vi "Compile Data Replay Loops.vi"(8 "error in (no error)":errorcluster, 10 "Channel Descriptors in":T1, 11 "Custom Device Ref":T11 format="%.0x") -> (0 "error out":errorcluster, 2 "Channel Descriptors out":T1, 3 "Custom Device Ref dup":T11 format="%.0x", 4 "DataReplayLoops":T9[](array[typedef]), 6 "DataReplayVoltages":T8[](array[typedef]))   [LabVIEW 2011, in "Engine Sim System Explorer.lvlib"]
uses:
  Engine Sim System Explorer.lvlib
  <vilib>/NI Veristand/Custom Device API/Custom Device Item Ref.ctl
  Shared/DataReplayLoopConfig.ctl
  Shared/DataReplayConfig.ctl
  Shared/DataReplayVoltageConfig.ctl
  Shared/Channel Descriptors.ctl
  Shared/FPGA Write Descriptor.ctl
  Shared/InputChannelTypes.ctl
  <vilib>/rvi/DataTransferAndStorage/Container/Common/niFpgaDataTypeControl.ctl
  Shared/FPGA Read Descriptor.ctl
  Shared/OutputChannelTypes.ctl
  Shared/Status Chan Descriptor.ctl
  Shared/Engine Simulation Global.vi
  <vilib>/NI Veristand/Custom Device Tools/Custom Device Utility Library/NI VeriStand - Search for All Items by GUID.vi
  <vilib>/NI Veristand/Custom Device API/Get Item Property (Double).vi
  <vilib>/rvi/Analysis/host/Private/Sample Rate To Loop Time (ticks).vi
  <vilib>/NI Veristand/Custom Device Tools/Custom Device Utility Library/Custom Device Utility Library.lvlib
  Engine Simulation Shared.lvlib
  <vilib>/rvi/Analysis/host/Public/NI_FpgaMspHost.lvlib
  <vilib>/NI Veristand/Custom Device API/Custom Device API.lvlib
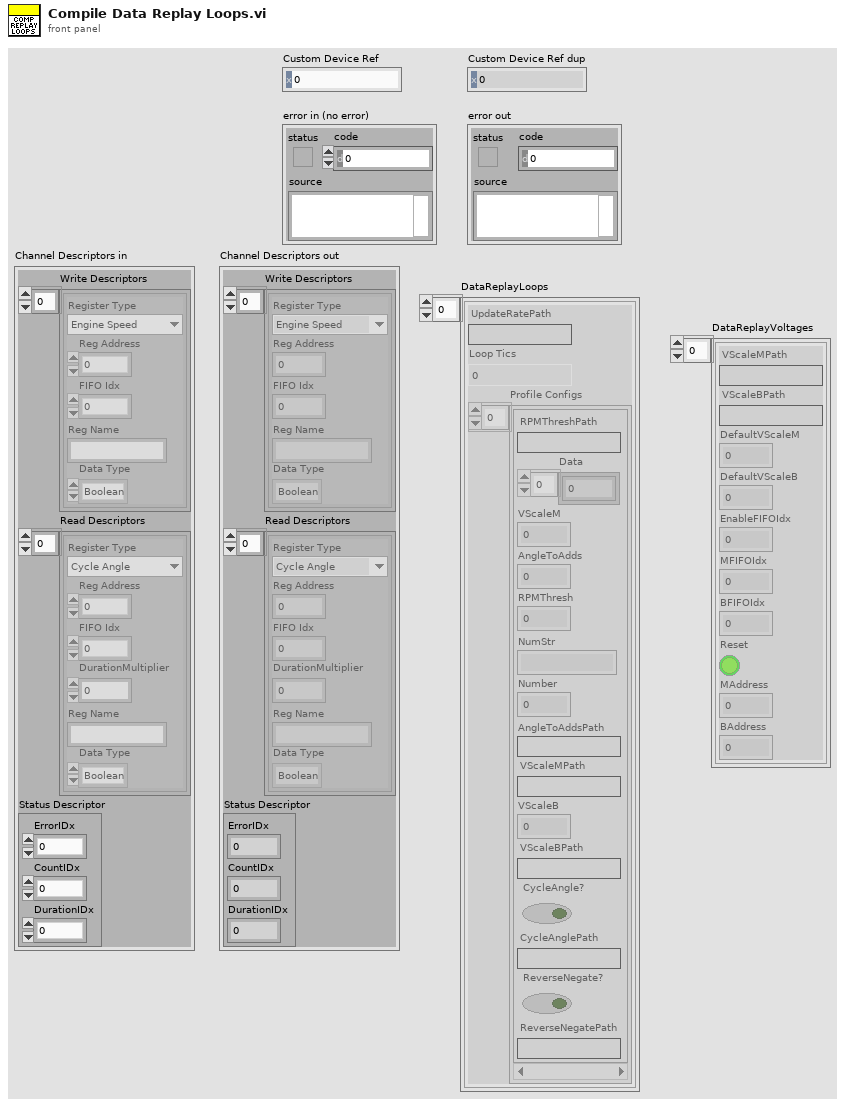
[diagram p1: front panel]
types:
  T1 = typedef "Engine Simulation Shared.lvlib/Channel Descriptors.ctl" = cluster{"Write Descriptors":T2[], "Read Descriptors":T5[], "Status Descriptor":T7}
  T2 = typedef "Engine Simulation Shared.lvlib/FPGA Write Descriptor.ctl" = cluster{"Register Type":T3, "Reg Address":u32, "FIFO Idx":i32, "Reg Name":string, "Data Type":T4}
  T3 = typedef "Engine Simulation Shared.lvlib/InputChannelTypes.ctl" = enum16{"Engine Speed", "Offset"}
  T4 = typedef "niFpgaDataTypeControl.ctl" = enum32{"Boolean", "I8", "I16", "I32", "I64", "U8", "U16", "U32", "U64", "FXP", "CustomControl"}
  T5 = typedef "Engine Simulation Shared.lvlib/FPGA Read Descriptor.ctl" = cluster{"Register Type":T6, "Reg Address":u32, "FIFO Idx":i32, "DurationMultiplier":dbl, "Reg Name":string, "Data Type":T4}
  T6 = typedef "Engine Simulation Shared.lvlib/OutputChannelTypes.ctl" = enum16{"Cycle Angle", "Crank Angle", "Time Duration", "Angle Duration", "Start Angle", "End Angle"}
  T7 = typedef "Engine Simulation Shared.lvlib/Status Chan Descriptor.ctl" = cluster{"ErrorIDx":i32, "CountIDx":i32, "DurationIDx":i32}
  T8 = typedef "Engine Simulation Shared.lvlib/DataReplayVoltageConfig.ctl" = cluster{"VScaleMPath":string, "VScaleBPath":string, "DefaultVScaleM":u32, "DefaultVScaleB":i32, "EnableFIFOIdx":i32, "MFIFOIdx":i32, "BFIFOIdx":i32, "Reset":bool, "MAddress":u32, "BAddress":u32}
  T9 = typedef "Engine Simulation Shared.lvlib/DataReplayLoopConfig.ctl" = cluster{"UpdateRatePath":string, "Loop Tics":u32, "Profile Configs":T10[]}
  T10 = typedef "Engine Simulation Shared.lvlib/DataReplayConfig.ctl" = cluster{"RPMThreshPath":string, "Data":i16[], "VScaleM":u32, "AngleToAdds":u32, "RPMThresh":u64, "NumStr":string, "Number":i8, "AngleToAddsPath":string, "VScaleMPath":string, "VScaleB":i32, "VScaleBPath":string, "CycleAngle?":bool, "CycleAnglePath":string, "ReverseNegate?":bool, "ReverseNegatePath":string}
  T11 = typedef "Custom Device API.lvlib/Custom Device Item Ref.ctl" = u64
  T12 = typedef "Custom Device API.lvlib/Custom Device Item Info.ctl" = cluster{"Name":string, "Is Channel":bool, "GUID":string}
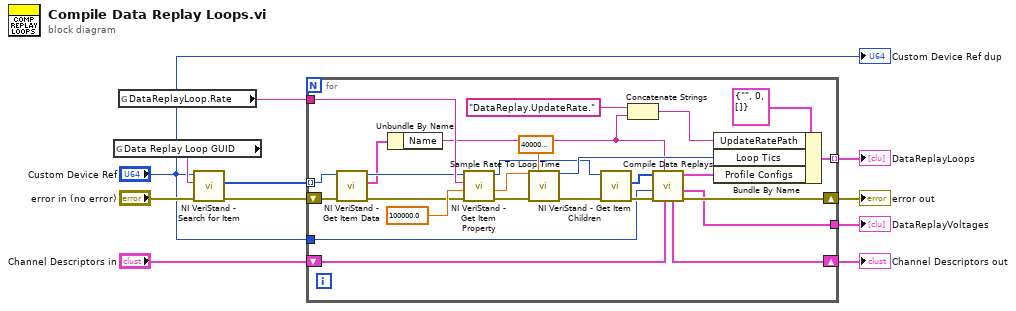
[diagram p0: block diagram]
diagram:
  n1 = global read "Engine Simulation Global.vi" "Data Replay Loop GUID"() -> (w10:string)
  n2 = global read "Engine Simulation Global.vi" "DataReplayLoop.Rate"() -> (w7:string)
  n3 = call-poly <vilib>:"NI VeriStand - Search for Item.vi"("error in"="error in (no error)", "Item GUID"=w10, "Section Ref in"="Custom Device Ref") -> ("error out"=w9:errorcluster, "Item Refs"=w8:T11[])  [unwired: 5 in, 2 out]
  n4 = for {
    shift-right: [w20] -> w6
    shift-left: w9 -> [w37]
    tunnel: w8 -> [w29] mode=indexing
    tunnel: w7 -> [w36]
    tunnel: [w23] -> w5 mode=indexing
    tunnel: [w15] -> w4
    tunnel: "Custom Device Ref" -> [w14]
    shift-right: [w12] -> w1
    shift-left: "Channel Descriptors in" -> [w13]
    n5 = call <vilib>:"NI VeriStand - Get Item Data.vi"("error in (no error)"=w37, "Item Ref in"=w29) -> ("error out"=w30:errorcluster, "Item Info"=w27:T12, "Item Ref out"=w28:T11)  [unwired: 6 in, 1 out]
    n6 = Unbundle By Name(w27) -> ("Name"=w16:string)
    n7 = call-poly <vilib>:"NI VeriStand - Get Item Property.vi"("error in (no error)"=w30, "Default Value"=100000.0, "Property Name"=w36, "Item Ref in"=w28) -> ("error out"=w34:errorcluster, "Value"=w33:dbl, "Item Ref out"=w24:T11)  [unwired: 4 in, 1 out]
    n8 = call-poly <vilib>:"Sample Rate To Loop Time.vi"("sample rate (S/s)"=w33, "FPGA clock rate (Hz)"=40000000.0, "error in (no error)"=w34) -> ("count (ticks/S)"=w26:u32, "error out"=w25:errorcluster)  [unwired: 10 in, 1 out]
    n9 = call <vilib>:"NI VeriStand - Get Item Children.vi"("error in (no error)"=w25, "Item Ref in"=w24) -> ("error out"=w22:errorcluster, "Child Refs"=w21:T11[])  [unwired: 6 in, 2 out]
    n10 = Concatenate Strings("DataReplay.UpdateRate." ("string"), w16) -> (w17:string)
    n11 = call "Compile Data Replays.vi"("Channel Descriptors in"=w13, "LoopName"=w16, "error in (no error)"=w22, "Custom Device Ref"=w14, "Data Replays Refs"=w21) -> ("error out"=w20:errorcluster, "DataReplayVoltages"=w15:T8[], "Data Replays"=w19:T10[], "Channel Descriptors out"=w12:T1)  [unwired: 3 in]
    n12 = Bundle By Name(cluster=T9 {"UpdateRatePath"="", "Loop Tics"=0, "Profile Configs"=[]} ("FullyCustom Config"), "UpdateRatePath"=w17, "Loop Tics"=w26, "Profile Configs"=w19) -> (w23:T9)
  }
  "error out" <- w6
  "DataReplayLoops" <- w5
  "DataReplayVoltages" <- w4
  "Channel Descriptors out" <- w1
  "Custom Device Ref dup" <- "Custom Device Ref"
